vi "Abort Reason.vi"(8 "error in (no error)":errorcluster) -> (0 "error out":errorcluster, 2 "Abort Reason Out":string)   [LabVIEW 2015]
panel:
  in  "OK Button":bool
  in  "Abort Reason":string="Operator Decision"
  out "Test Sequence":i32(listbox)=-2
  # "Test Aborted"
  # "Please enter the reason the test was aborted"
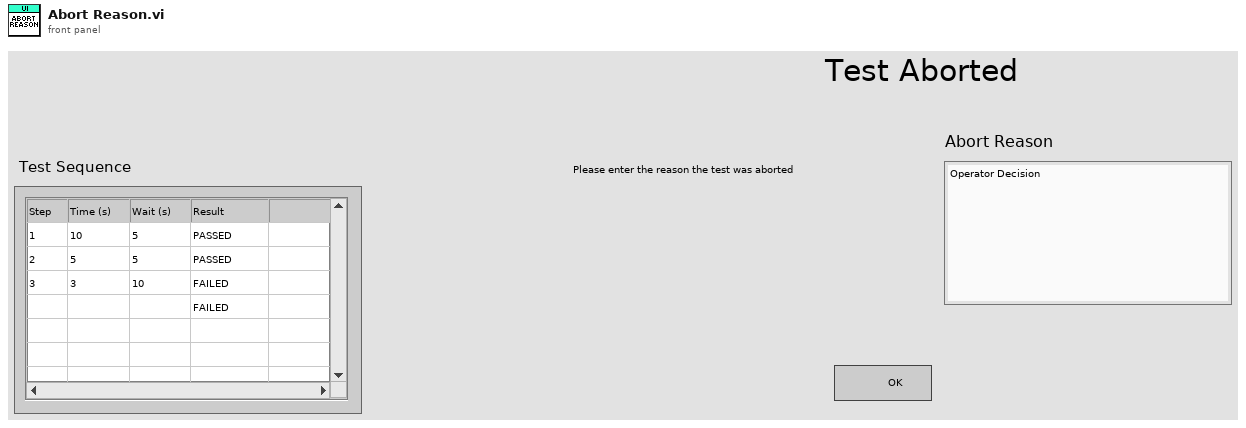
[diagram p1: front panel]
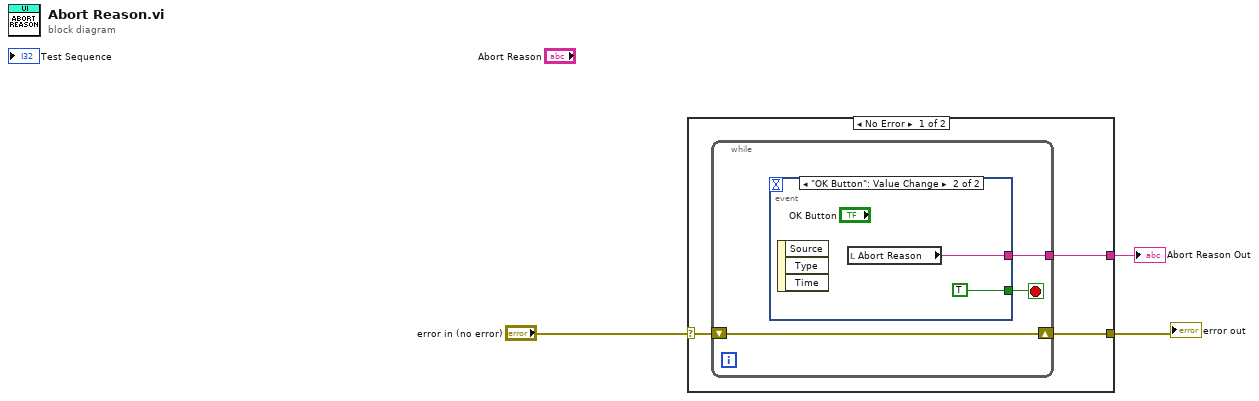
[diagram p0: block diagram]
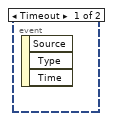
[diagram p2: hidden frame]
diagram:
  n1 = case shown="No Error" "error in (no error)" {
    selector: "error in (no error)" -> [w5 w12]
    tunnel: [w6 _] -> w3
    tunnel: [w4 w12] -> w2
    frame No Error {
      n2 = while {
        tunnel: [w8] -> w6
        shift-right: [w7] -> w4
        shift-left: w5 -> [w7]
        stop <- w9 stop-if-true
        n3 = event shown="[1] \"OK Button\": Value Change" {
          selector: _ -> [_ _]
          dyn-events: _ -> [_ _]
          timeout: _ -> [_ _]
          tunnel: [_ TRUE] -> w9
          tunnel: [_ w10] -> w8
          event Timeout {
            n4 = event-data() -> ()  [unwired: 1 in, 3 out]
          }
          event "OK Button": Value Change {
            n5 = event-data() -> ()  [unwired: 1 in, 3 out]
            n6 = local read "Abort Reason"() -> (w10:string)
          }
        }
      }
    }
    frame Error {
    }
  }
  "error out" <- w2
  "Abort Reason Out" <- w3
